vi "Write ColumnSizes.vi"(8 "error in (no error)":errorcluster, 10 "ColumnSizes":i32[](array[numeric]), 11 "AdjustableMulticolumnListbox in":refnum<class "AdjMCLB.lvclass">) -> (0 "error out":errorcluster, 3 "AdjustableMulticolumnListbox out":refnum<class "AdjMCLB.lvclass">)   [LabVIEW 2020, in "AdjMCLB.lvclass"]
uses:
  AdjMCLB.lvclass
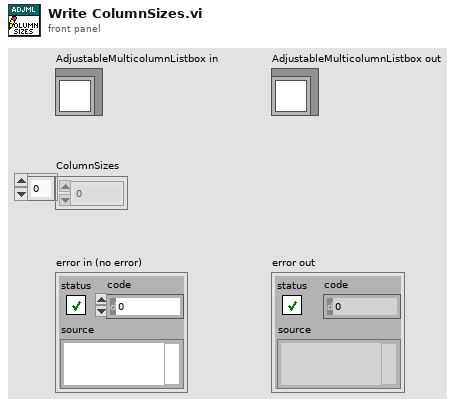
[diagram p1: front panel]
types:
  T1 = typedef "AdjustableMulticolumnListbox.lvclass/State Data.ctl" = cluster{"FitControlToPane?":bool, "ColumnSizes":i32[]}
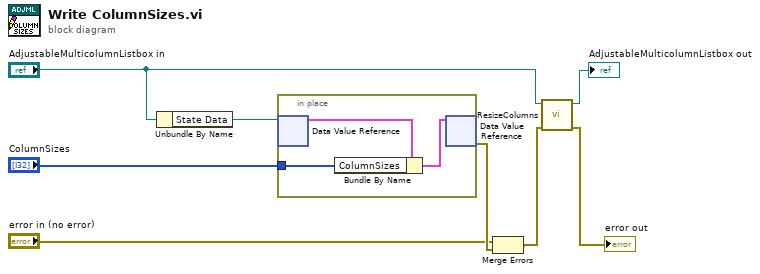
[diagram p0: block diagram]
diagram:
  n1 = Unbundle By Name("AdjustableMulticolumnListbox in") -> ("State Data"=w8:refnum<data-value>)
  n2 = in-place {
    in-place-border: "ColumnSizes" -> [w9]
    n3 = in-place-dvr #1(w8) -> (w11:T1)  [unwired: 1 out]
    n4 = Bundle By Name(cluster=w11, "ColumnSizes"=w9) -> (w10:T1)
    n5 = in-place-dvr #1(w10) -> (w7:errorcluster)  [unwired: 1 out]
  }
  n6 = Merge Errors("error in (no error)", w7) -> (w2:errorcluster)
  n7 = call "ResizeColumns.vi"("error in (no error)"=w2, "AdjustableMulticolumnListbox in"="AdjustableMulticolumnListbox in") -> ("error out"=→"error out":errorcluster, "AdjustableMulticolumnListbox out"=→"AdjustableMulticolumnListbox out":refnum<class "AdjMCLB.lvclass">)  [unwired: 8 in]
